vi "DIO_PWM_Encoder.vi"(0 "DIO.1:0.OUT":fxp<+,2,2> format="%.0b", 1 "DIO.1:0.DIR":fxp<+,2,2> format="%.0b", 3 "PWM.GROUP IN":T1 {"PWM.1.CNFG" format="%08b"; "PWM.0.CNFG" format="%08b"}, 4 "Encoder.GROUP IN":T2 {"ENC.STAT" format="%08b"}, 6 "DIO0/PWM0/ENC.A Refnum":refnum<k21>, 7 "DIO.1:0.Selector":fxp<+,4,4> format="%.0b", 8 "DIO1/PWM1/ENC.B Refnum":refnum<k21>) -> (14 "IN 1:0":fxp<+,2,2> format="%02b", 17 "PWM.GROUP OUT":T1 {"PWM.1.CNFG" format="%08b"; "PWM.0.CNFG" format="%08b"}, 18 "Encoder.GROUP OUT":T2 {"ENC.STAT" format="%08b"})   [LabVIEW 2019]
uses:
  Utilities/PWM Configuration Group.ctl
  Utilities/Encoder Configuration Group.ctl
panel:
  # "This VI switches between the DIO functionality and the PWM/Encoder/I2C functionality for the specified FPGA I/O channels. Each bit has a selector which contains two-bits booleans.\n- If SELECT 0 is 00, DIO enabled.\n- If SELECT 0 is 01, PWM enabled.\n- If SELECT 0 is 10, Encoder enabled.\n- If SELECT 0 is 11, I2C enabled."
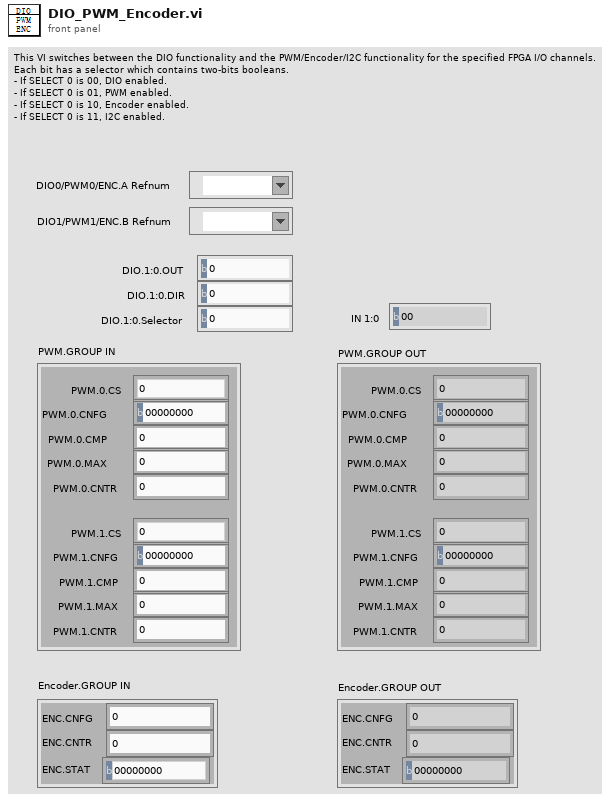
[diagram p1: front panel]
types:
  T1 = typedef "PWM Configuration Group.ctl" = cluster{"PWM.0.CS":u8, "PWM.0.CNFG":u8, "PWM.0.CMP":u16, "PWM.0.MAX":u16, "PWM.0.CNTR":u16, "PWM.1.CS":u8, "PWM.1.CNFG":u8, "PWM.1.CMP":u16, "PWM.1.MAX":u16, "PWM.1.CNTR":u16}
  T2 = typedef "Encoder Configuration Group.ctl" = cluster{"ENC.CNFG":u8, "ENC.CNTR":u32, "ENC.STAT":u8}
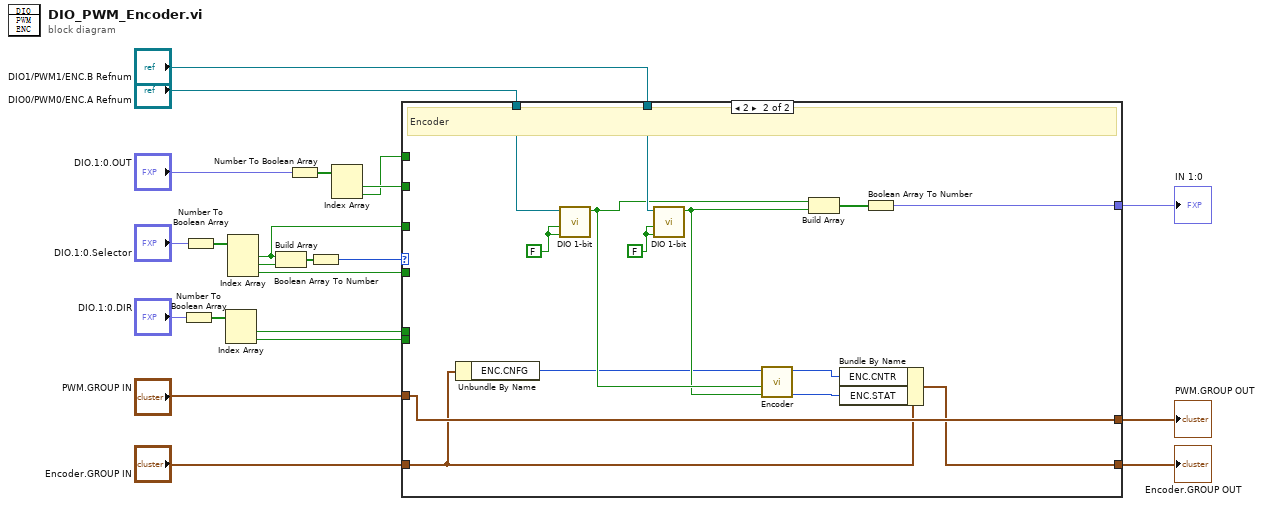
[diagram p0: block diagram]
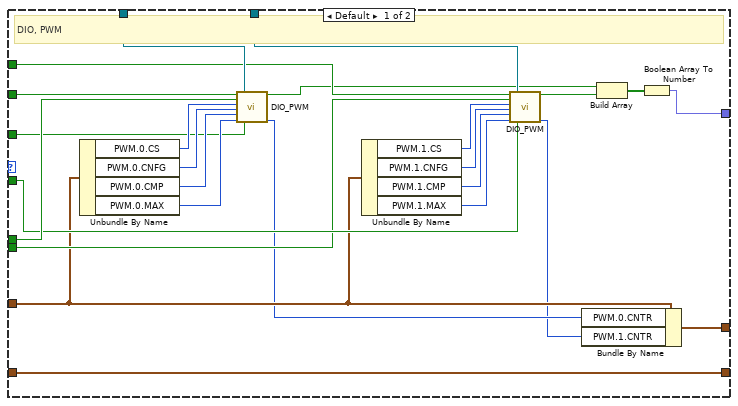
[diagram p2: hidden frame]
diagram:
  n1 = Number To Boolean Array(number="DIO.1:0.DIR") -> (Boolean array=w19:bool[])
  n2 = Number To Boolean Array(number="DIO.1:0.Selector") -> (Boolean array=w21:bool[])
  n3 = Index Array(array=w19) -> (element #1=w13:bool, element #2=w12:bool)  [unwired: 2 in]
  n4 = Index Array(array=w21) -> (element #1=w1:bool, element #2=w17:bool, element #3=w2:bool)  [unwired: 3 in]
  n5 = Build Array(w1, w17) -> (w16:bool[])
  n6 = Number To Boolean Array(number="DIO.1:0.OUT") -> (Boolean array=w20:bool[])
  n7 = Boolean Array To Number(Boolean array=w16) -> (number=w7:u8)
  n8 = Index Array(array=w20) -> (element #1=w15:bool, element #2=w14:bool)  [unwired: 2 in]
  n9 = case shown="2" w7 {
    tunnel: w15 -> [w44 _]
    tunnel: w14 -> [w35 _]
    tunnel: w13 -> [w43 _]
    tunnel: w12 -> [w34 _]
    tunnel: "PWM.GROUP IN" -> [w33 w61]
    tunnel: "Encoder.GROUP IN" -> [w46 w50]
    tunnel: [w47 w61] -> w8
    tunnel: [w46 w49] -> w3
    tunnel: [w23 w58] -> w6
    tunnel: "DIO0/PWM0/ENC.A Refnum" -> [w45 w57]
    tunnel: "DIO1/PWM1/ENC.B Refnum" -> [w37 w56]
    tunnel: w2 -> [w36 _]
    tunnel: w1 -> [w38 _]
    frame Default {
      # "DIO, PWM"
      n10 = Unbundle By Name(w33) -> ("PWM.0.CS"=w42:u8, "PWM.0.CNFG"=w41:u8, "PWM.0.CMP"=w40:u16, "PWM.0.MAX"=w39:u16)
      n11 = call "DIO_PWM.vi"("DIO.OUT"=w44, "DIO.DIR"=w43, "PWM.CS"=w42, "PWM.CNFG"=w41, "PWM.CMP"=w40, "PWM.MAX"=w39, "DIO/PWM"=w45, "SELECT"=w38) -> ("DIO.IN"=w26:bool, "PWM.CNTR"=w28:u16)  [unwired: 10 in]
      n12 = Unbundle By Name(w33) -> ("PWM.1.CS"=w32:u8, "PWM.1.CNFG"=w31:u8, "PWM.1.CMP"=w30:u16, "PWM.1.MAX"=w29:u16)
      n13 = call "DIO_PWM.vi"("DIO.OUT"=w35, "DIO.DIR"=w34, "PWM.CS"=w32, "PWM.CNFG"=w31, "PWM.CMP"=w30, "PWM.MAX"=w29, "DIO/PWM"=w37, "SELECT"=w36) -> ("DIO.IN"=w25:bool, "PWM.CNTR"=w27:u16)  [unwired: 10 in]
      n14 = Bundle By Name(cluster=w33, "PWM.0.CNTR"=w28, "PWM.1.CNTR"=w27) -> (w47:T1)
      n15 = Build Array(w26, w25) -> (w24:bool[])
      n16 = Boolean Array To Number(Boolean array=w24) -> (number=w23:fxp<+,2,2>)
    }
    frame 2 {
      w52 = FALSE ("DIR")
      w53 = FALSE ("DIR")
      # "Encoder"
      n17 = Unbundle By Name(w50) -> ("ENC.CNFG"=w51:u8)
      n18 = call "DIO 1-bit.vi"("DIR"=w53, "OUT"=w53, "DIO Refnum"=w57) -> ("IN"=w55:bool)  [unwired: 8 in]
      n19 = call "DIO 1-bit.vi"("DIR"=w52, "OUT"=w52, "DIO Refnum"=w56) -> ("IN"=w54:bool)  [unwired: 8 in]
      n20 = call "Encoder.vi"("Phase B"=w54, "Phase A"=w55, "CNFG"=w51) -> ("STAT"=w48:u8, "CNTR"=w60:u32)  [unwired: 7 in]
      n21 = Build Array(w55, w54) -> (w59:bool[])
      n22 = Bundle By Name(cluster=w50, "ENC.CNTR"=w60, "ENC.STAT"=w48) -> (w49:T2)
      n23 = Boolean Array To Number(Boolean array=w59) -> (number=w58:fxp<+,2,2>)
    }
  }
  "IN 1:0" <- w6
  "PWM.GROUP OUT" <- w8
  "Encoder.GROUP OUT" <- w3
